vi "Create.vi"(10 "Logs":string[](array[string])) -> (3 "Logs List Value out":refnum<class "Logs List Value.lvclass">)   [LabVIEW 2020, in "VolatusData.lvlib" / "Logs List Value.lvclass"]
uses:
  Logs List Value.lvclass
  Logs List Value.lvclass/Logs List Value.ctl
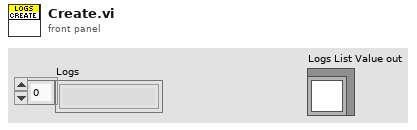
[diagram p1: front panel]
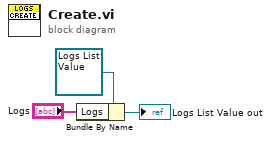
[diagram p0: block diagram]
diagram:
  n1 = Bundle By Name(cluster=refnum<class "Logs List Value.lvclass"> refnum ("Logs List Value out"), "Logs"="Logs") -> (→"Logs List Value out":refnum<class "Logs List Value.lvclass">)
